vi "read default menu name.vi"(8 "error in":errorcluster, 11 "CVT Engine Editor in":refnum<class "CVT Engine Editor.lvclass">) -> (0 "error out":errorcluster, 2 "default menu name":string, 3 "CVT Engine Editor out":refnum<class "CVT Engine Editor.lvclass">)   [LabVIEW 2013, in "CVT Engine Editor.lvclass"]
uses:
  CVT Engine Editor.lvclass
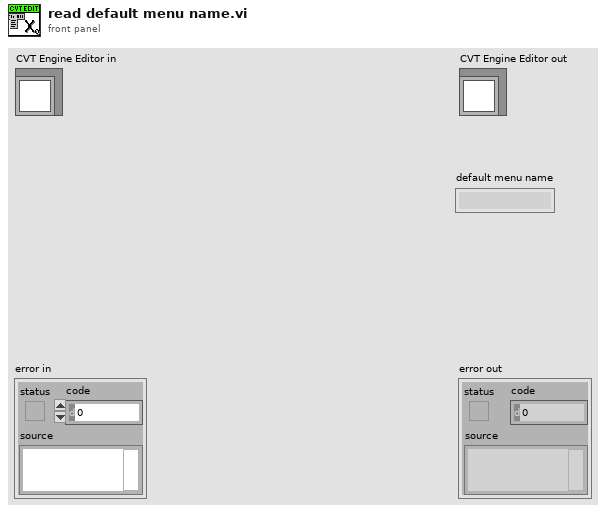
[diagram p1: front panel]
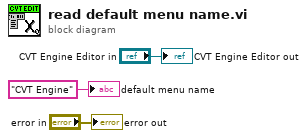
[diagram p0: block diagram]
diagram:
  "error out" <- "error in"
  "CVT Engine Editor out" <- "CVT Engine Editor in"
  "default menu name" <- "CVT Engine" ("default menu name")
